vi "LineM.vi"(5 "Yin":dbl, 7 "Xin":dbl, 8 "Y2":dbl, 9 "X2":dbl, 10 "Y1":dbl, 11 "X1":dbl) -> (0 "Yout":dbl, 1 "Xout":dbl, 2 "Ydistance":dbl, 3 "Xdistance":dbl, 4 "m":dbl)   [LabVIEW 2019]
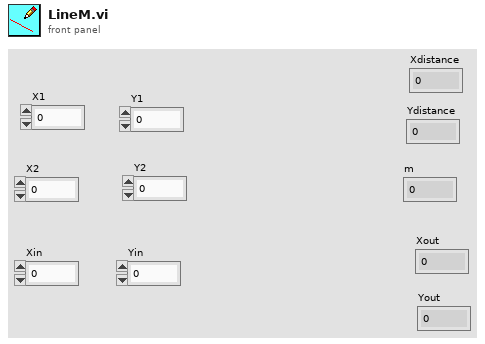
[diagram p1: front panel]
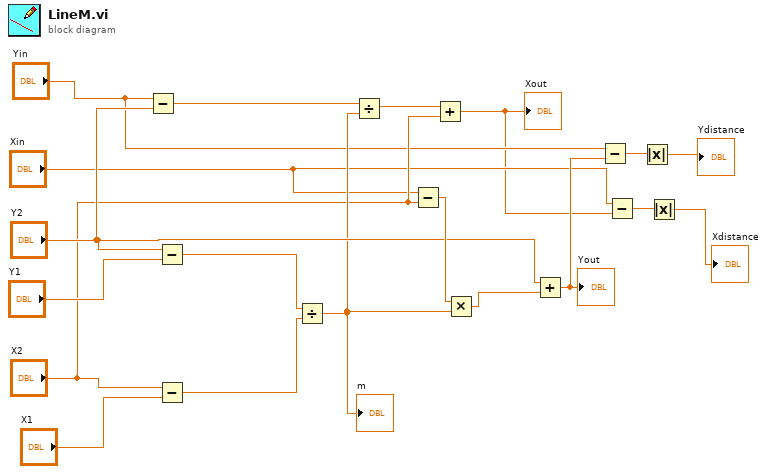
[diagram p0: block diagram]
diagram:
  n1 = Subtract(x="Yin", y="Y2") -> (x-y=w12:dbl)
  n2 = Subtract(x="Y2", y="Y1") -> (x-y=w17:dbl)
  n3 = Subtract(x="X2", y="X1") -> (x-y=w16:dbl)
  n4 = Divide(x=w17, y=w16) -> (x/y=w11:dbl)
  "m" <- w11
  n5 = Divide(x=w12, y=w11) -> (x/y=w10:dbl)
  n6 = Subtract(x="Xin", y="X2") -> (x-y=w15:dbl)
  n7 = Add(x=w10, y="X2") -> (x+y=w2:dbl)
  "Xout" <- w2
  n8 = Multiply(x=w15, y=w11) -> (x*y=w14:dbl)
  n9 = Add(x="Y2", y=w14) -> (x+y=w7:dbl)
  "Yout" <- w7
  n10 = Subtract(x="Yin", y=w7) -> (x-y=w6:dbl)
  n11 = Subtract(x="Xin", y=w2) -> (x-y=w4:dbl)
  n12 = Absolute Value(x=w6) -> (abs(x)=→"Ydistance":dbl)
  n13 = Absolute Value(x=w4) -> (abs(x)=→"Xdistance":dbl)
